vi "NIRFSG_Initialize.vi"(8 "error in (no error)":errorcluster, 10 "Reset?":bool, 11 "RFSG Handle":refnum<k15>) -> (0 "error out":errorcluster)   [LabVIEW 2015]
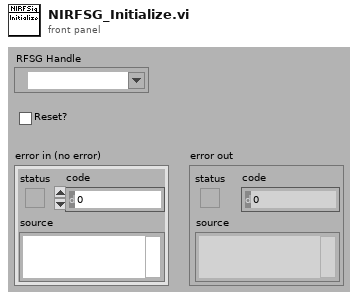
[diagram p1: front panel]
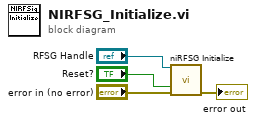
[diagram p0: block diagram]
diagram:
  n1 = call <instrlib>:"niRFSG Initialize.vi"("resource name"="RFSG Handle", "reset device"="Reset?", "error in"="error in (no error)") -> ("error out"=→"error out":errorcluster)  [unwired: 11 in, 1 out]
